vi "Set_possition.vi"(8 "error in (no error)":errorcluster, 10 "possition(rev)":dbl, 11 "Motor in":refnum<class "Motor.lvclass">) -> (0 "error out":errorcluster, 3 "Motor out":refnum<class "Motor.lvclass">)   [LabVIEW 2019, in "Motor.lvclass"]
uses:
  Motor.lvclass
  Motor.lvclass/Motor.ctl
  Motor Serial class/Serial.lvclass
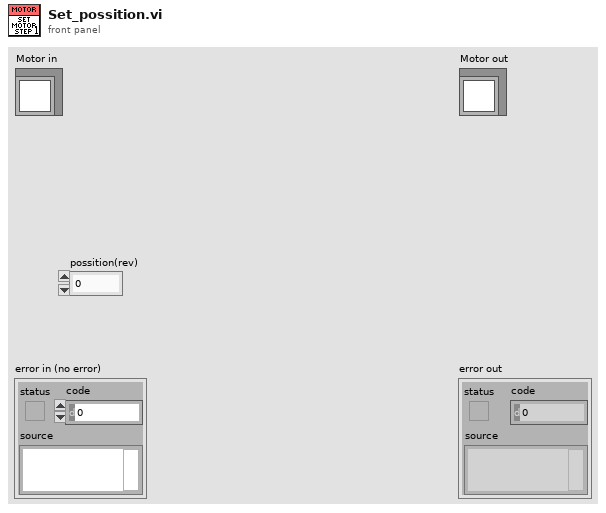
[diagram p1: front panel]
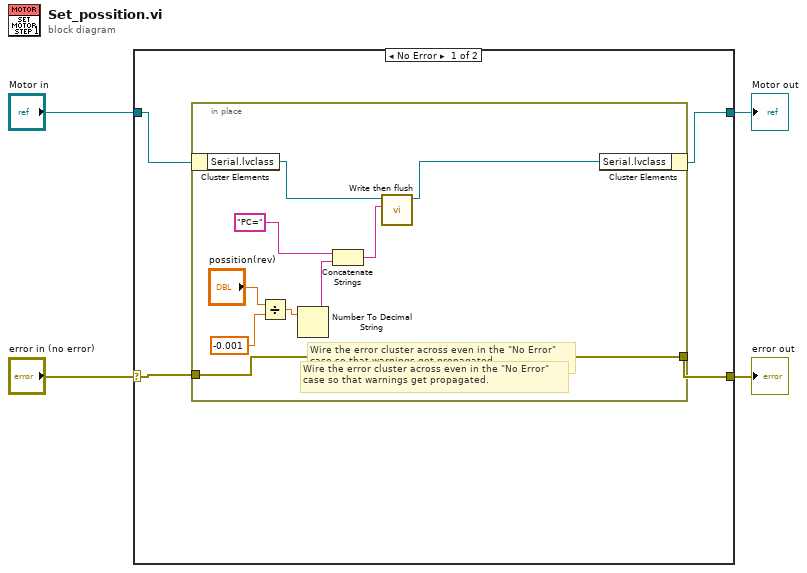
[diagram p0: block diagram]
diagram:
  n1 = case shown="No Error" "error in (no error)" {
    selector: "error in (no error)" -> [w8 w19]
    tunnel: [w7 w19] -> w3
    tunnel: [w6 w18] -> w1
    tunnel: "Motor in" -> [w5 w18]
    frame No Error {
      # "Wire the error cluster across even in the \"No Error\"\ncase so that warnings get propagated."
      n2 = in-place {
        in-place-border: w8 -> [w17]
        in-place-border: [w17] -> w7
        # "Wire the error cluster across even in the \"No Error\"\ncase so that warnings get propagated."
        n3 = in-place-cluster #1(w5) -> ("Serial.lvclass"=w16:refnum<class "Serial.lvclass">)
        n4 = Divide(x="possition(rev)", y=-0.001) -> (x/y=w10:dbl)
        n5 = Number To Decimal String(number=w10) -> (decimal integer string=w9:string)  [unwired: 1 in]
        n6 = Concatenate Strings("PC=" ("string"), w9) -> (w13:string)
        n7 = call "Write then flush.vi"("TX Data"=w13, "Motor_Serial in"=w16) -> ("Motor_Serial out"=w15:refnum<class "Serial.lvclass">)  [unwired: 8 in, 1 out]
        n8 = in-place-cluster #1("Serial.lvclass"=w15) -> (w6:refnum<class "Motor.lvclass">)
      }
    }
    frame Error {
    }
  }
  "error out" <- w3
  "Motor out" <- w1
